vi "SystemLink_Write_String.vi"(9 "String":string, 11 "SL_XControl":T1(xcontrol)) -> ()   [LabVIEW 2019]
uses:
  SL_XControl.xctl
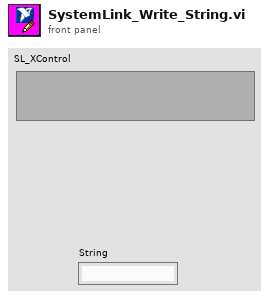
[diagram p1: front panel]
types:
  T1 = cluster{"Tag":string, "Type":string, "Data":string}
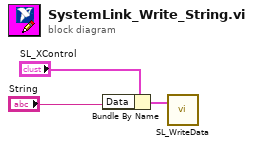
[diagram p0: block diagram]
diagram:
  n1 = Bundle By Name(cluster="SL_XControl", "Data"="String") -> (w1:T1)
  n2 = call "SL_WriteData.vi"("Tag"=w1) -> ()  [unwired: 11 in]
